vi "Read From Connection.vi"(8 "error in (no error)":errorcluster, 9 "Timeout (ms)":i32, 10 "Bytes to Read":i32, 11 "Connection Reference In":refnum<data-value>) -> (0 "error out":errorcluster, 1 "TimeOut?":bool, 2 "Data":string, 3 "Connection Reference Out":refnum<data-value>)   [LabVIEW 2020, in "Connection Reference.lvlib" / "Connection Reference.lvclass"]
uses:
  <vilib>/gpm_packages/@cs/Network-interface/Source/Connection Reference/Connection Reference/Connection Reference.lvclass
  <vilib>/gpm_packages/@cs/Network-interface/Source/Connection Reference/Connection Reference/Connection Reference.lvclass/Connection Reference.ctl
  <vilib>/gpm_packages/@cs/Network-interface/Source/Connection Reference/IConnection/IConnection.lvclass
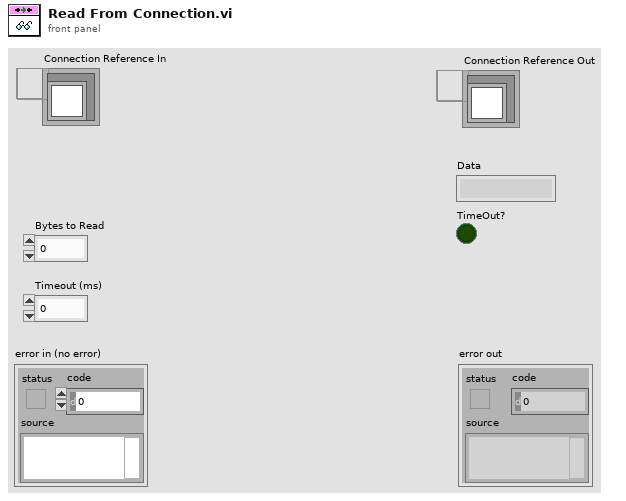
[diagram p1: front panel]
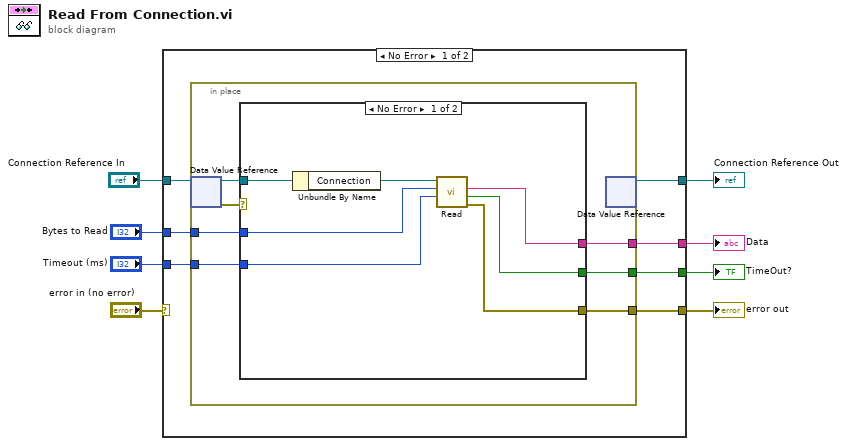
[diagram p0: block diagram]
diagram:
  n1 = case shown="No Error" "error in (no error)" {
    selector: "error in (no error)" -> [_ w31]
    tunnel: "Connection Reference In" -> [w15 w32]
    tunnel: [w14 w32] -> w7
    tunnel: [w13 w31] -> w5
    tunnel: "Bytes to Read" -> [w12 _]
    tunnel: "Timeout (ms)" -> [w11 _]
    tunnel: [w10 _] -> w2
    tunnel: [w9 _] -> w1
    frame No Error {
      n2 = in-place {
        in-place-border: [w20] -> w13
        in-place-border: w12 -> [w19]
        in-place-border: w11 -> [w18]
        in-place-border: [w17] -> w10
        in-place-border: [w16] -> w9
        n3 = in-place-dvr #1(w15) -> (w22:refnum<class "Connection Reference.lvclass">, w21:errorcluster)
        n4 = case shown="No Error" w21 {
          selector: w21 -> [_ w30]
          tunnel: w22 -> [w23 _]
          tunnel: [w29 w30] -> w20
          tunnel: w19 -> [w28 _]
          tunnel: w18 -> [w27 _]
          tunnel: [w26 _] -> w17
          tunnel: [w25 _] -> w16
          frame No Error {
            n5 = Unbundle By Name(w23) -> ("Connection"=w24:refnum<class "IConnection.lvclass">)
            n6 = call-dynamic "Read.vi"("Timeout (ms)"=w27, "Bytes to Read"=w28, "IConnection in"=w24) -> ("error out"=w29:errorcluster, "TimeOut?"=w26:bool, "Data"=w25:string)  [unwired: 5 in, 1 out]
          }
          frame Error {
            # "#todo add useful error here"
          }
        }
        n7 = in-place-dvr #1() -> (w14:refnum<data-value>)  [unwired: 1 in, 1 out]
      }
    }
    frame Error {
    }
  }
  "error out" <- w5
  "Connection Reference Out" <- w7
  "TimeOut?" <- w2
  "Data" <- w1
